vi "example test.vi"() -> ()   [LabVIEW 2013, in "Modbus Slave tests.lvlib"]
doc: "Platypus Framework 1.0.1.65\nNI Systems Engineering - National Instruments"
uses:
  Modbus Slave tests.lvlib
  configuration/Modbus Slave configuration.lvclass
  execution/Modbus Slave runtime.lvclass
  module channel/Modbus Module Channel.lvclass
  <vilib>/NI/Tag Bus/tag/Data Type.ctl
  <vilib>/NI/Tag Bus/tag/tag descriptor.lvclass
  <vilib>/NI/Tag Bus Module Framework/channel/channel classification.ctl
  <vilib>/NI/Tag Bus Module Framework/channel/TBM channel.lvclass
  module channel/data bank type.ctl
  <vilib>/NI/Tag Bus/table/data table.lvlib
  <vilib>/NI/Tag Bus/table/data polymorphs/write one/write Double.vi
  <vilib>/NI/Tag Bus/table/data polymorphs/read one/read Double.vi
  <vilib>/NI/Tag Bus/table/data polymorphs/read one/read Boolean.vi
  <vilib>/NI/Tag Bus/table/data polymorphs/write one/write Boolean.vi
  <vilib>/NI/Modbus Library/API/Wrapper/API Main.lvlib
  <vilib>/NI/Modbus Library/API/Wrapper/Create TCP Master.vi
  <vilib>/NI/Modbus Library/API/Master/Modbus Master.lvclass
panel:
  out "D out":bool
  out "B out":dbl
  in  "C in":bool
  in  "A in":dbl
  in  "stop 2":bool
  out "C":bool
  in  "D":bool
  out "A":dbl
  in  "B":dbl
  in  "stop":bool
  out "final error":errorcluster
  out "output error":errorcluster
  out "input error":errorcluster
  out "init error":errorcluster
  out "correct execution settings":bool
  out "serialization problem":errorcluster
  out "invalid configuration":errorcluster
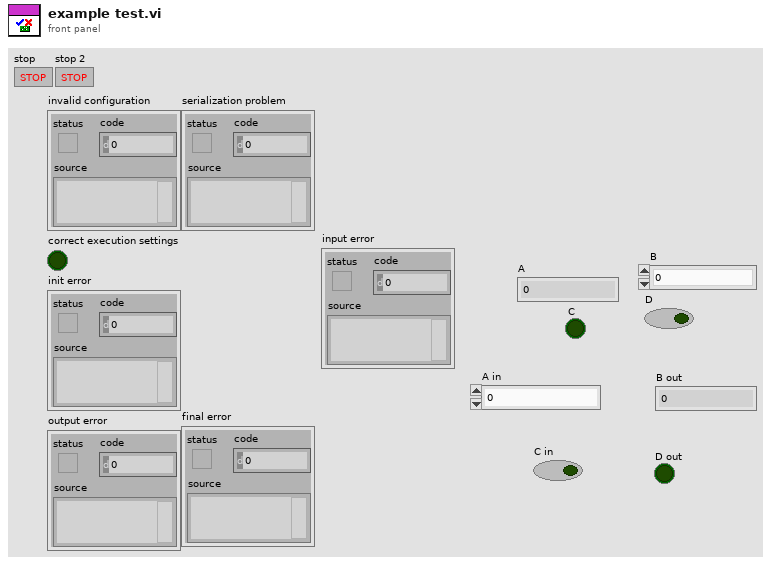
[diagram p1: front panel]
types:
  T1 = typedef "Modbus Module Channel.lvclass/data bank type.ctl" = enum16{"coils", "discrete inputs", "input registers", "holding registers"}
  T2 = typedef "TBM channel.lvclass/channel classification.ctl" = enum16{"input data", "output data", "processing parameter", "processing result"}
  T3 = typedef "tag bus.lvlib/tag descriptor.lvclass/Data Type.ctl" = enum16{"Double", "Single", "I64", "I32", "I16", "I8", "U64", "U32", "U16", "U8", "Boolean", "String", "Array of Double", "Array of Single", "Array of I64", "Array of I32", "Array of I16", "Array of I8", "Array of U64", "Array of U32", "Array of U16", "Array of U8", "Array of Boolean", "Array of String"}
  T4 = typedef "TBM channel.lvclass/data tables.ctl" = cluster{"input data":T5, "processing parameter":T5, "processing result":T5, "output data":T5}
  T5 = typedef "tag bus.lvlib/dictionary table pair.ctl" = cluster{"data dictionary":refnum<class "data dictionary.lvclass">, "data table":T6}
  T6 = typedef "tag bus.lvlib/data table.lvlib/data table.ctl" = cluster{"Double":dbl[], "Single":sgl[], "I64":i64[], "I32":i32[], "I16":i16[], "I8":i8[], "U64":u64[], "U32":u32[], "U16":u16[], "U8":u8[], "Boolean":bool[], "String":string[], "Array of Double":cluster{"DBL Array":dbl[]}[], "Array of Single":cluster{"SGL Array":sgl[]}[], "Array of I64":cluster{"I64 Array":i64[]}[], "Array of I32":cluster{"I32 Array":i32[]}[], "Array of I16":cluster{"I16 Array":i16[]}[], "Array of I8":cluster{"I8 Array":i8[]}[], "Array of U64":cluster{"U64 Array":u64[]}[], "Array of U32":cluster{"U32 Array":u32[]}[], "Array of U16":cluster{"U16 Array":u16[]}[], "Array of U8":cluster{"U8 Array":u8[]}[], "Array of Boolean":cluster{"Boolean Array":bool[]}[], "Array of String":cluster{"String Array":string[]}[]}
  T7 = typedef "TBM module execution interface.lvclass/execution settings.ctl" = cluster{"reads inputs":bool, "processes data":bool, "writes outputs":bool}
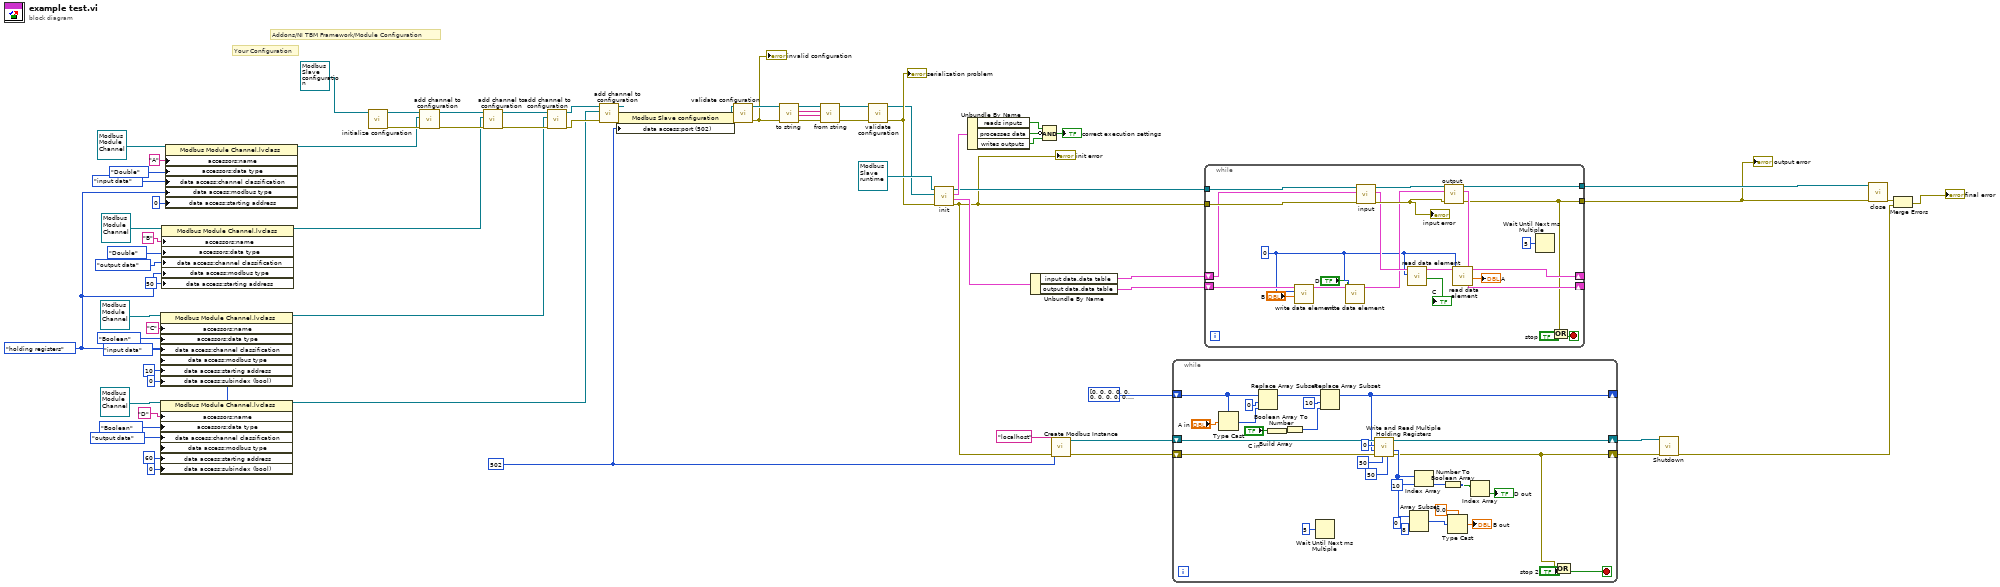
[diagram p0: block diagram]
diagram:
  w9 = u16 502 ("port (502)")
  w18 = data_bank_type."holding registers" ("modbus type")
  # "Your Configuration"
  # "Addons/NI TBM Framework/Module Configuration"
  n1 = property class="Modbus Module Channel.lvclass"(reference=refnum<class "Modbus Module Channel.lvclass"> refnum ("Modbus Module Channel.lvclass"), "accessors:name"="C" ("name"), "accessors:data type"=Data_Type."Boolean" ("data type"), "data access:channel classification"=channel_classification."input data" ("channel classification"), "data access:modbus type"=w18, "data access:starting address"=u16 10 ("starting address"), "data access:subindex (bool)"=0 ("subindex (bool)")) -> (reference out=w37:refnum<class "Modbus Module Channel.lvclass">)  [unwired: 1 in, 1 out]
  n2 = property class="Modbus Module Channel.lvclass"(reference=refnum<class "Modbus Module Channel.lvclass"> refnum ("Modbus Module Channel.lvclass"), "accessors:name"="D" ("name"), "accessors:data type"=Data_Type."Boolean" ("data type"), "data access:channel classification"=channel_classification."output data" ("channel classification"), "data access:modbus type"=w18, "data access:starting address"=u16 60 ("starting address"), "data access:subindex (bool)"=0 ("subindex (bool)")) -> (reference out=w38:refnum<class "Modbus Module Channel.lvclass">)  [unwired: 1 in, 1 out]
  n3 = property class="Modbus Module Channel.lvclass"(reference=refnum<class "Modbus Module Channel.lvclass"> refnum ("Modbus Module Channel.lvclass"), "accessors:name"="B" ("name"), "accessors:data type"=Data_Type."Double" ("data type"), "data access:channel classification"=channel_classification."output data" ("channel classification"), "data access:modbus type"=w18, "data access:starting address"=u16 50 ("starting address")) -> (reference out=w36:refnum<class "Modbus Module Channel.lvclass">)  [unwired: 1 in, 1 out]
  n4 = property class="Modbus Module Channel.lvclass"(reference=refnum<class "Modbus Module Channel.lvclass"> refnum ("Modbus Module Channel.lvclass"), "accessors:name"="A" ("name"), "accessors:data type"=Data_Type."Double" ("data type"), "data access:channel classification"=channel_classification."input data" ("channel classification"), "data access:modbus type"=w18, "data access:starting address"=u16 0 ("starting address")) -> (reference out=w35:refnum<class "Modbus Module Channel.lvclass">)  [unwired: 1 in, 1 out]
  n5 = call-dynamic "initialize configuration.vi"("configuration in"=refnum<class "Modbus Slave configuration.lvclass"> refnum ("tag bus configurable plugin module configuration")) -> ("error out"=w49:errorcluster, "configuration out"=w50:refnum<class "Modbus Slave configuration.lvclass">)  [unwired: 8 in, 1 out]
  n6 = call "add channel to configuration.vi"("error in"=w49, "Modbus Module Channel.lvclass"=w35, "Modbus Slave configuration in"=w50) -> ("error out"=w51:errorcluster, "Modbus Slave configuration out"=w45:refnum<class "Modbus Slave configuration.lvclass">)  [unwired: 7 in]
  n7 = call "add channel to configuration.vi"("error in"=w51, "Modbus Module Channel.lvclass"=w36, "Modbus Slave configuration in"=w45) -> ("error out"=w46:errorcluster, "Modbus Slave configuration out"=w44:refnum<class "Modbus Slave configuration.lvclass">)  [unwired: 7 in]
  n8 = call "add channel to configuration.vi"("error in"=w46, "Modbus Module Channel.lvclass"=w37, "Modbus Slave configuration in"=w44) -> ("error out"=w48:errorcluster, "Modbus Slave configuration out"=w42:refnum<class "Modbus Slave configuration.lvclass">)  [unwired: 7 in]
  n9 = call "add channel to configuration.vi"("error in"=w48, "Modbus Module Channel.lvclass"=w38, "Modbus Slave configuration in"=w42) -> ("error out"=w43:errorcluster, "Modbus Slave configuration out"=w11:refnum<class "Modbus Slave configuration.lvclass">)  [unwired: 7 in]
  n10 = property class="Modbus Slave configuration"(reference=w11, error in=w43, "data access:port (502)"=w9) -> (reference out=w10:refnum<class "Modbus Slave configuration.lvclass">, error out=w12:errorcluster)
  n11 = call-dynamic "validate configuration.vi"("error in"=w12, "Modbus Slave configuration in"=w10) -> ("error out"=w72:errorcluster, "Modbus Slave configuration out"=w73:refnum<class "Modbus Slave configuration.lvclass">)  [unwired: 8 in]
  "invalid configuration" <- w72
  n12 = call-dynamic "to string.vi"("error in"=w72, "Modbus Slave configuration in"=w73) -> ("error out"=w68:errorcluster, "data"=w69:string, "version"=w70:string, "Modbus Slave configuration out"=w71:refnum<class "Modbus Slave configuration.lvclass">)  [unwired: 6 in]
  n13 = call-dynamic "from string.vi"("error in"=w68, "data"=w69, "version"=w70, "Modbus Slave configuration in"=w71) -> ("error out"=w66:errorcluster, "Modbus Slave configuration out"=w67:refnum<class "Modbus Slave configuration.lvclass">)  [unwired: 6 in]
  n14 = call-dynamic "validate configuration.vi"("error in"=w66, "Modbus Slave configuration in"=w67) -> ("error out"=w64:errorcluster, "Modbus Slave configuration out"=w63:refnum<class "Modbus Slave configuration.lvclass">)  [unwired: 8 in]
  "serialization problem" <- w64
  n15 = call-dynamic "init.vi"("error in"=w64, "TBM module configuration in"=w63, "Modbus Slave runtime in"=refnum<class "Modbus Slave runtime.lvclass"> refnum ("tag bus configurable plugin module")) -> ("error out"=w13:errorcluster, "data allocations"=w57:T4, "execution settings"=w62:T7, "Modbus Slave runtime out"=w56:refnum<class "Modbus Slave runtime.lvclass">)  [unwired: 5 in]
  "init error" <- w13
  n16 = Unbundle By Name(w62) -> ("reads inputs"=w59:bool, "processes data"=w61:bool, "writes outputs"=w60:bool)
  n17 = Unbundle By Name(w57) -> ("input data.data table"=w15:T6, "output data.data table"=w14:T6)
  n18 = Compound Arithmetic op=AND(w59, invert w61, w60) -> (→"correct execution settings":bool)
  n19 = call-poly <vilib>:"Create Modbus Instance.vi"("error in"=w13, "port (502)"=w9, "address"="localhost") -> ("error out"=w6:errorcluster, "TCP master instance"=w7:refnum<class "Modbus Master.lvclass">)  [unwired: 7 in]
  n20 = while {
    shift-right: [w98] -> w3
    shift-left: w7 -> [w100]
    shift-right: [w74] -> w4
    shift-left: w6 -> [w99]
    shift-right: [w94] -> _
    shift-left: u16[] [0, 0, 0, 0, 0, 0, 0, 0, 0, 0, 0, 0, 0, 0, 0, 0, 0, 0, 0, 0, 0, 0, 0, 0, 0, 0, 0, 0, 0, 0, 0, 0, 0, 0, 0, 0, 0, 0, 0, 0, 0, 0, 0, 0, 0, 0, 0, 0, 0, 0] ("write values") -> [w89]
    stop <- w101 stop-if-true
    n21 = Type Cast(type=w89, x="A in") -> (*(type *) &x=w88:u16[])
    n22 = Replace Array Subset(array=w89, new element=w88, index=0) -> (w93:u16[])
    n23 = Build Array("C in") -> (w86:bool[])
    n24 = Boolean Array To Number(Boolean array=w86) -> (number=w85:u16)
    n25 = Wait Until Next ms Multiple(millisecond multiple=u32 5) -> ()  [unwired: 1 out]
    n26 = Replace Array Subset(array=w93, new element=w85, index=10) -> (w94:u16[])
    n27 = call-dynamic "Write and Read Multiple Holding Registers.vi"("read count"=u16 50, "read starting address"=u16 50, "error in"=w99, "write values"=w94, "write starting address"=u16 0, "Modbus instance in"=w100) -> ("error out"=w74:errorcluster, "read values"=w79:u16[], "Modbus instance out"=w98:refnum<class "Modbus Master.lvclass">)  [unwired: 3 in]
    n28 = Array Subset(array=w79, index=0, length=8) -> (w82:u16[])
    n29 = Index Array(array=w79, index=10) -> (element=w77:u16)
    n30 = Number To Boolean Array(number=w77) -> (Boolean array=w76:bool[])
    n31 = Type Cast(type=0.0, x=w82) -> (*(type *) &x=→"B out":dbl)
    n32 = Index Array(array=w76) -> (element=→"D out":bool)  [unwired: 1 in]
    n33 = Or(x=w74, y="stop 2") -> (x .or. y?=w101:bool)
  }
  n34 = while {
    tunnel: w56 -> [w125]
    tunnel: [w123] -> w55
    tunnel: [w104] -> w54
    tunnel: w13 -> [w122]
    shift-right: [w113] -> _
    shift-left: w15 -> [w120]
    shift-right: [w117] -> _
    shift-left: w14 -> [w119]
    stop <- w105 stop-if-true
    w111 = 0 ("index")
    n35 = call-poly <vilib>:"write data element.vi"("value"="B", "index"=w111, "data table in"=w119) -> ("data table out"=w115:T6)  [unwired: 8 in]
    n36 = call-poly <vilib>:"write data element.vi"("value"="D", "index"=w111, "data table in"=w115) -> ("data table out"=w114:T6)  [unwired: 8 in]
    n37 = call-dynamic "input.vi"("error in"=w122, "data table in"=w120, "Modbus Slave runtime in"=w125) -> ("error out"=w118:errorcluster, "data table out"=w116:T6, "Modbus Slave runtime out"=w124:refnum<class "Modbus Slave runtime.lvclass">)  [unwired: 6 in]
    "input error" <- w118
    n38 = call-poly <vilib>:"read data element.vi"("index"=w111, "data table in"=w116) -> ("value"=→"C":bool, "data table out"=w112:T6)  [unwired: 8 in]
    n39 = call-dynamic "output.vi"("error in"=w118, "data table in"=w114, "Modbus Slave runtime in"=w124) -> ("error out"=w104:errorcluster, "data table out"=w117:T6, "Modbus Slave runtime out"=w123:refnum<class "Modbus Slave runtime.lvclass">)  [unwired: 6 in]
    n40 = call-poly <vilib>:"read data element.vi"("index"=w111, "data table in"=w112) -> ("value"=→"A":dbl, "data table out"=w113:T6)  [unwired: 8 in]
    n41 = Wait Until Next ms Multiple(millisecond multiple=u32 5) -> ()  [unwired: 1 out]
    n42 = Or(x=w104, y="stop") -> (x .or. y?=w105:bool)
  }
  "output error" <- w54
  n43 = call-dynamic "Shutdown.vi"("error in"=w4, "Modbus master in"=w3) -> ("error out"=w2:errorcluster)  [unwired: 9 in]
  n44 = call-dynamic "close.vi"("error in"=w54, "Modbus Slave runtime in"=w55) -> ("error out"=w53:errorcluster)  [unwired: 9 in]
  n45 = Merge Errors(w53, w2) -> (→"final error":errorcluster)
